vi "Remove Topic.vi"(8 "error in (no error)":errorcluster, 10 "Topic":refnum<class "Topic.lvclass">, 11 "TopicLookupTable":refnum<data-value>) -> (0 "error out":errorcluster, 3 "TopicLookupTable":refnum<data-value>)   [LabVIEW 2015, in "Mediator.lvlib" / "TopicLookupTable.lvclass"]
doc: "<License>\nCopyright © 2017 Composed Systems, LLC | All rights reserved\nwww.composed.io\n\nAuthor: Ethan Stern <ethan.stern@composed.io>\n\nThis software is provided \"AS IS\" WITHOUT WARRANTIES, either express or implied, AND IS FOR EDUCATIONAL PURPOSES ONLY.\n</License>"
uses:
  TopicLookupTable.lvclass
  Topic/Topic.lvclass
  TopicLookupTable.lvclass/TopicLookupTable.ctl
  Topic/Topic.lvclass/Topic.ctl
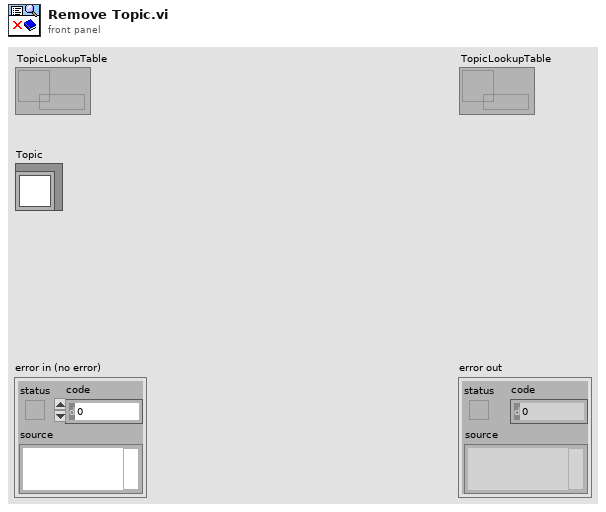
[diagram p1: front panel]
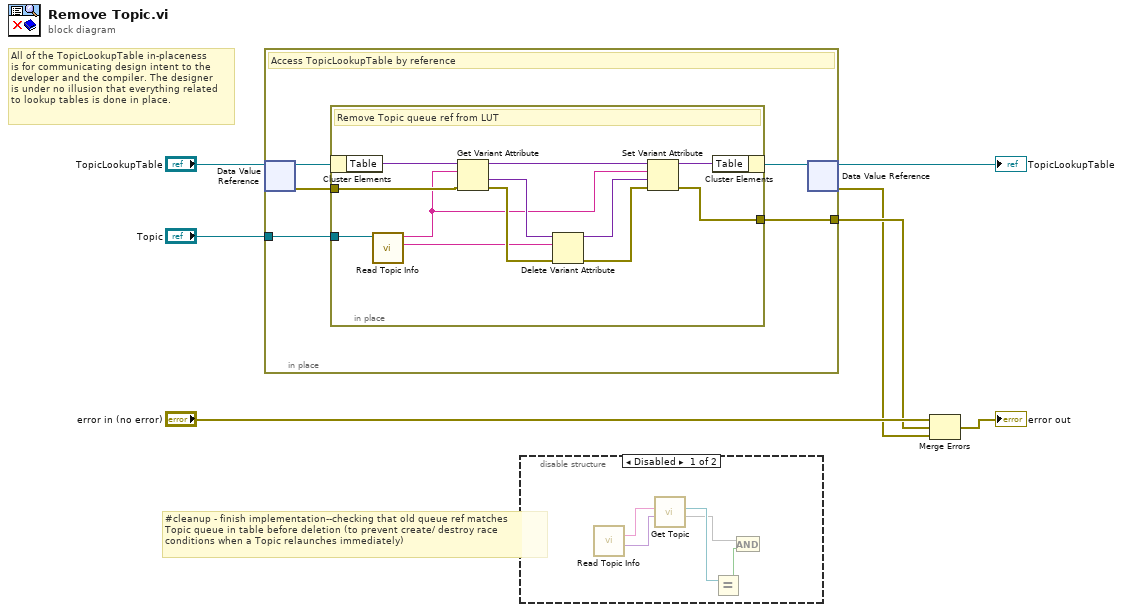
[diagram p0: block diagram]
diagram:
  # "#cleanup - finish implementation--checking that old queue ref matches\nTopic queue in table before deletion (to prevent create/ destroy race\nconditions when a Topic relaunches immediately)"
  # "All of the TopicLookupTable in-placeness\nis for communicating design intent to the\ndeveloper and the compiler. The designer\nis under no illusion that everything related\nto lookup tables is done in place."
  n1 = in-place {
    in-place-border: [w12] -> w5
    in-place-border: "Topic" -> [w11]
    # "Access TopicLookupTable by reference"
    n2 = in-place-dvr #1("TopicLookupTable") -> (w10:refnum<class "TopicLookupTable.lvclass">, w8:errorcluster)
    n3 = in-place {
      in-place-border: [w21] -> w12
      in-place-border: w11 -> [w13]
      in-place-border: w8 -> [w23]
      # "Remove Topic queue ref from LUT"
      n4 = in-place-cluster #2(w10) -> ("Table"=w20:variant)
      n5 = call "Read Topic Info.vi"("Topic in"=w13) -> ("Name"=w15:string, "Type"=w14:string)  [unwired: 7 in, 2 out]
      n6 = Get Variant Attribute(Variant=w20, name=w14, error in=w23) -> (duplicate Variant=w19:variant, value=w18:variant, error out=w24:errorcluster)  [unwired: 1 in, 1 out]
      n7 = Delete Variant Attribute(4:w24, 6:w15, 7:w18) -> (0:w16:errorcluster, 3:w17:variant)  [unwired: 1 out]
      n8 = Set Variant Attribute(Variant=w19, name=w14, value=w17, error in=w16) -> (Variant out=w22:variant, error out=w21:errorcluster)  [unwired: 1 out]
      n9 = in-place-cluster #2("Table"=w22) -> (w9:refnum<class "TopicLookupTable.lvclass">)
    }
    n10 = in-place-dvr #1(w9) -> (→"TopicLookupTable":refnum<data-value>, w2:errorcluster)
  }
  n11 = disable-structure shown="Disabled" {
    frame Disabled {
      n12 = call "Read Topic Info.vi"() -> ("Last Topic Value"=w29:variant, "Name"=w30:string)  [unwired: 8 in, 2 out]
      n13 = call "Get Topic.vi"("Topic Type"=w29, "Topic Name"=w30) -> (1:w25, "Topic Refnum"=w28:refnum<class "Message Enqueuer.lvclass">, 3:"TopicLookupTable"=w31:refnum<data-value>, 11:"TopicLookupTable"=w32:refnum<data-value>)  [unwired: 5 in, 1 out]
      n14 = Equal?(x=w28) -> (y=w27:refnum<class "Message Enqueuer.lvclass">, x = y?=w26:bool)
      n15 = And(x=w25, y=w26) -> ()  [unwired: 1 out]
    }
    frame Enabled {
    }
  }
  n16 = Merge Errors("error in (no error)", w5, w2) -> (→"error out":errorcluster)
